vi "ReadEyeFileFast_I8.vi"(0 "new file path":path=path "C:/WINDOWS/DESKTOP/rri.eye", 6 "Header format":u16(ring) items=["Riverside Format", "Ron Linear"]) -> (9 "Digitizer (dB)":sgl, 10 "new path out":path, 11 "RF Att":sgl format="%.2f", 12 "# A/D bits":i32, 13 "2-D data array":i8[][](array[numeric]), 14 "# lines per scan":i32, 15 "# rf points per line":u16, 16 "sample rate MHz":u16, 17 "sector scan angle":sgl format="%.2f", 18 "delay":sgl format="%.2f", 19 "pivot distance":sgl format="%.2f")   [LabVIEW 2022 SP3]
panel:
  out "Votage scaling":T1
  out "error out":errorcluster
  out "Head length":i16
  out "file size (bytes)":i32
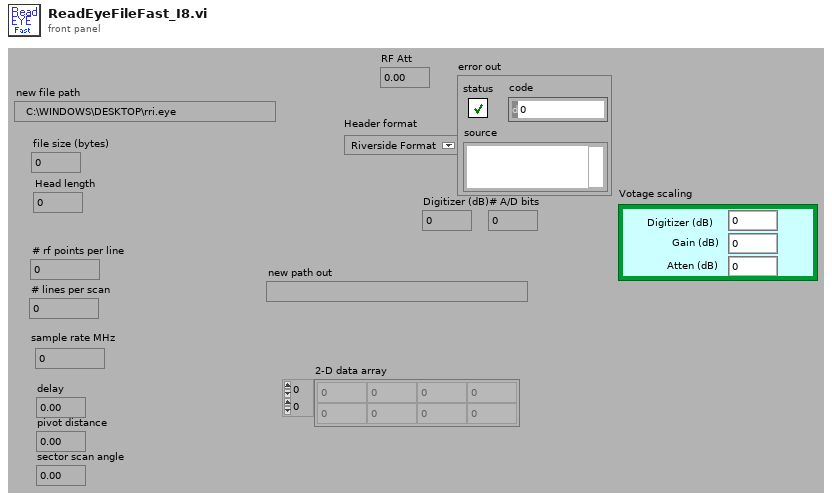
[diagram p1: front panel]
types:
  T1 = cluster{"Digitizer (dB)":sgl, "Gain (dB)":sgl, "Atten (dB)":sgl}
  T2 = typedef "Header.ctl" = cluster{"header info":cluster{"Header":string, "Head length":i16}, "A/D info":cluster{"# rf points per line":u16, "# lines per scan":u16, "sample rate MHz":u16, "# A/D bits":i16, "# bytes per A/D":u16, "TGC Flag":u16, "A/D Type":string}, "Tranducer Info":cluster{"bandwidth":sgl, "center freq":sgl, "start freq":sgl, "ID":i32}, "Scan Info":cluster{"delay":sgl, "pivot distance":sgl, "sector scan angle":sgl, "operator":string, "Scan Mode":string, "location":string}, "Time/Date Info":cluster{"date":string, "time":string}, "RF Info":cluster{"RF file name":string, "RF file att":string, "RF cal file name":string, "RF cal file att":string}, "Patient Info":cluster{"ID":string, "extended ID":string, "age":u16, "sex":string, "previously\nscanned":string, "PSA":sgl, "LOS":u8, "Ethnicty 2":u8, "Race":u8}, "Tissue Type":cluster{"organ":i16, "disease type":i16, "disease location":i16, "IQ_pts":u16, "RcvBuffer":u8, "RcvFrame":u16, "IQBuff":u8, "IQFrame":u16, "IQPage":u8}, "Votage scaling":cluster{"Digitizer (dB)":sgl, "Gain (dB)":sgl, "Atten (dB)":sgl}, "Comment":string, "Misc Info":cluster{"avg num":u16, "c speed":i16, "Div By or SF zones":i16, "XMIT CHS":u8, "RCV CHS":u8, "Xmit angle":sgl}, "Therapy Parameters":cluster{"Theraputic Freq (MHz)":sgl, "Time on (s)":sgl, "Therapy amplitude (mV)":sgl, "Lines Before":u16, "Lines After":u16}, "Scan Settings":cluster{"Energy (uJ or V)":u8, "Damp (Ohm) or Fc":u8, "HP Filt (KHz)":u8, "LP Filt (MHz)":u8, "Gain (db)":u8, "prf (kHz)":sgl, "Distance between\nscan lines (um)":u16, "Distance between\nscan planes (um)":u16, "Scan line gap (um)":sgl, "Scan plane gap (um)":sgl}, "Compression Parameters":cluster{"F1 (MHz)":sgl, "F2 (MHz)":sgl, "% taper":sgl, "duration":sgl}, "Patient Info Xtra":cluster{"First Name":string, "Last Name":string, "Notes":string}, "ROI Box":u16[]}
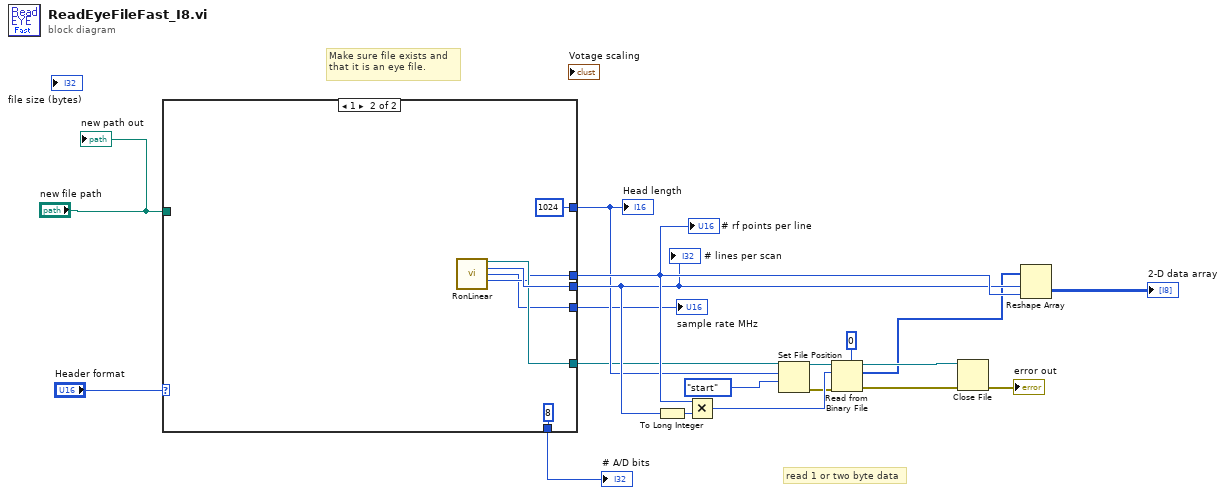
[diagram p0: block diagram]
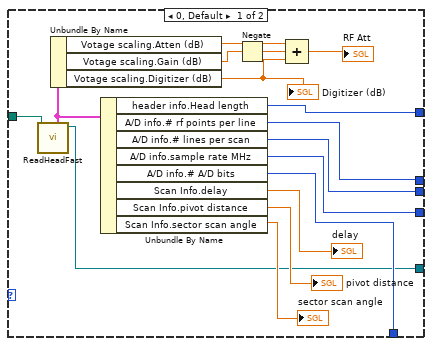
[diagram p2: hidden frame]
diagram:
  # "Make sure file exists and that it is an eye file."
  # "read 1 or two byte data"
  n1 = case shown="1" "Header format" {
    tunnel: [w33 w37] -> w15
    tunnel: [w32 w41] -> w14
    tunnel: [w21 w40] -> w10
    tunnel: [w34 i16 1024] -> w11
    tunnel: [w31 8] -> w5
    tunnel: "new file path" -> [w35 _]
    tunnel: [w20 w36] -> w1
    frame 0, Default {
      n2 = call "ReadHeadFast.vi"("new file path"=w35) -> ("refnum out"=w21:refnum<file>, "Header In"=w22:T2)  [unwired: 7 in, 2 out]
      n3 = Unbundle By Name(w22) -> ("Votage scaling.Atten (dB)"=w25:sgl, "Votage scaling.Gain (dB)"=w26:sgl, "Votage scaling.Digitizer (dB)"=w27:sgl)
      "Digitizer (dB)" <- w27
      n4 = Unbundle By Name(w22) -> ("header info.Head length"=w34:i16, "A/D info.# rf points per line"=w33:u16, "A/D info.# lines per scan"=w32:u16, "A/D info.sample rate MHz"=w20:u16, "A/D info.# A/D bits"=w31:i16, "Scan Info.delay"=→"delay":sgl, "Scan Info.pivot distance"=→"pivot distance":sgl, "Scan Info.sector scan angle"=→"sector scan angle":sgl)
      n5 = Negate(x=w26) -> (-x=w23:sgl)
      n6 = Compound Arithmetic op=ADD(w25, w23, w27) -> (→"RF Att":sgl)
    }
    frame 1 {
      n7 = call "RonLinear.vi"() -> ("refnum out"=w40:refnum<file>, "# lines per scan"=w41:i32, "sample rate"=w36:u16, "# rf points per line"=w37:u16)  [unwired: 1 in, 11 out]
    }
  }
  "# rf points per line" <- w15
  "Head length" <- w11
  "# lines per scan" <- w14
  "sample rate MHz" <- w1
  "# A/D bits" <- w5
  n8 = To Long Integer(number=w14) -> (32bit integer=w17:i32)
  n9 = Multiply(x=w15, y=w17) -> (x*y=w18:i32)
  n10 = Set File Position(offset (in bytes) (0)=w11, refnum=w10, from (0:start)=enum16{"start", "end", "current"}."start" ("pos mode (0:2)")) -> (refnum out=w3:refnum<file>, error out=w2:errorcluster)  [unwired: 1 in]
  n11 = Read from Binary File(5:i8 0, 8:w2, 10:w18, 11:w3) -> (0:w8:errorcluster, 2:w12:i8[], 3:w13:refnum<file>)  [unwired: 3 out]
  n12 = Close File(refnum=w13, error in=w8) -> (error out=→"error out":errorcluster)  [unwired: 1 out]
  n13 = Reshape Array(w12, w14, w15) -> (→"2-D data array":i8[][])
  "new path out" <- "new file path"
